vi "FPFA v4.vi"() -> ()   [LabVIEW 2015]
uses:
  <vilib>/Instr/_visa.llb/VISA Configure Serial Port (Instr).vi
  MFC1/inc/ThorZStepper.lvlib
panel:
  in  "Delay (s)":u32=1 min=1 step=1
  in  "# scan":u32=1 min=1 step=1
  in  "Autofocus":bool
  out "MFC1":bool
  out "Scan Enable":bool
  out "Current ZPos (mm)":dbl
  in  "Shutter":bool
  in  "MFC1 control":bool
  out "Scan finished":bool
  out "Elapsed Time (s)":dbl
  in  "# of measurment":i32=1
  out "Curr Well":cluster{"Row":u16, "Column":u16}={"Row"=1, "Column"=1} {"Column" items=["1", "2", "3", "4", "5", "6", "7", "8", "9", "10", "11", "12"]; "Row" items=["A", "B", "C", "D", "E", "F", "G", "H"]}
  in  "Set zero":bool
  in  "Abort":bool
  in  "Collection time":dbl=150.0 caption="s"
  in  "MoveWell":bool
  in  "Column":u16(ring)=1 items=["1", "2", "3", "4", "5", "6", "7", "8", "9", "10", "11", "12"]
  in  "Row":u16(ring)=1 items=["A", "B", "C", "D", "E", "F", "G", "H"]
  in  "Scan":bool
  in  "Move Abs":bool
  in  "YAbs":dbl caption="YAbs (micron)"
  in  "XAbs":dbl caption="XAbs (micron)"
  out "Response":string
  in  "Command":string
  out "error out":errorcluster
  in  "Send cmd":bool
  out "XPos":dbl
  out "YPos":dbl
  in  "Calibration":bool
  in  "stop":bool
  out "StageMoved":bool
  in  "Port":i32=5
  # "Move to Well"
  # "Stage Location"
  # "Move Absolute"
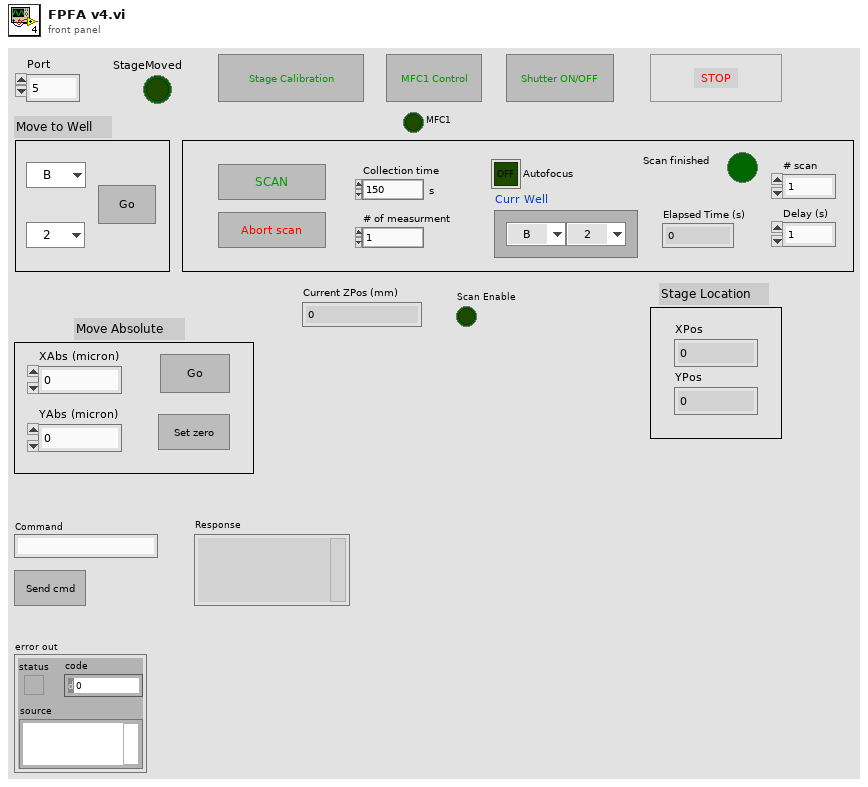
[diagram p1: front panel]
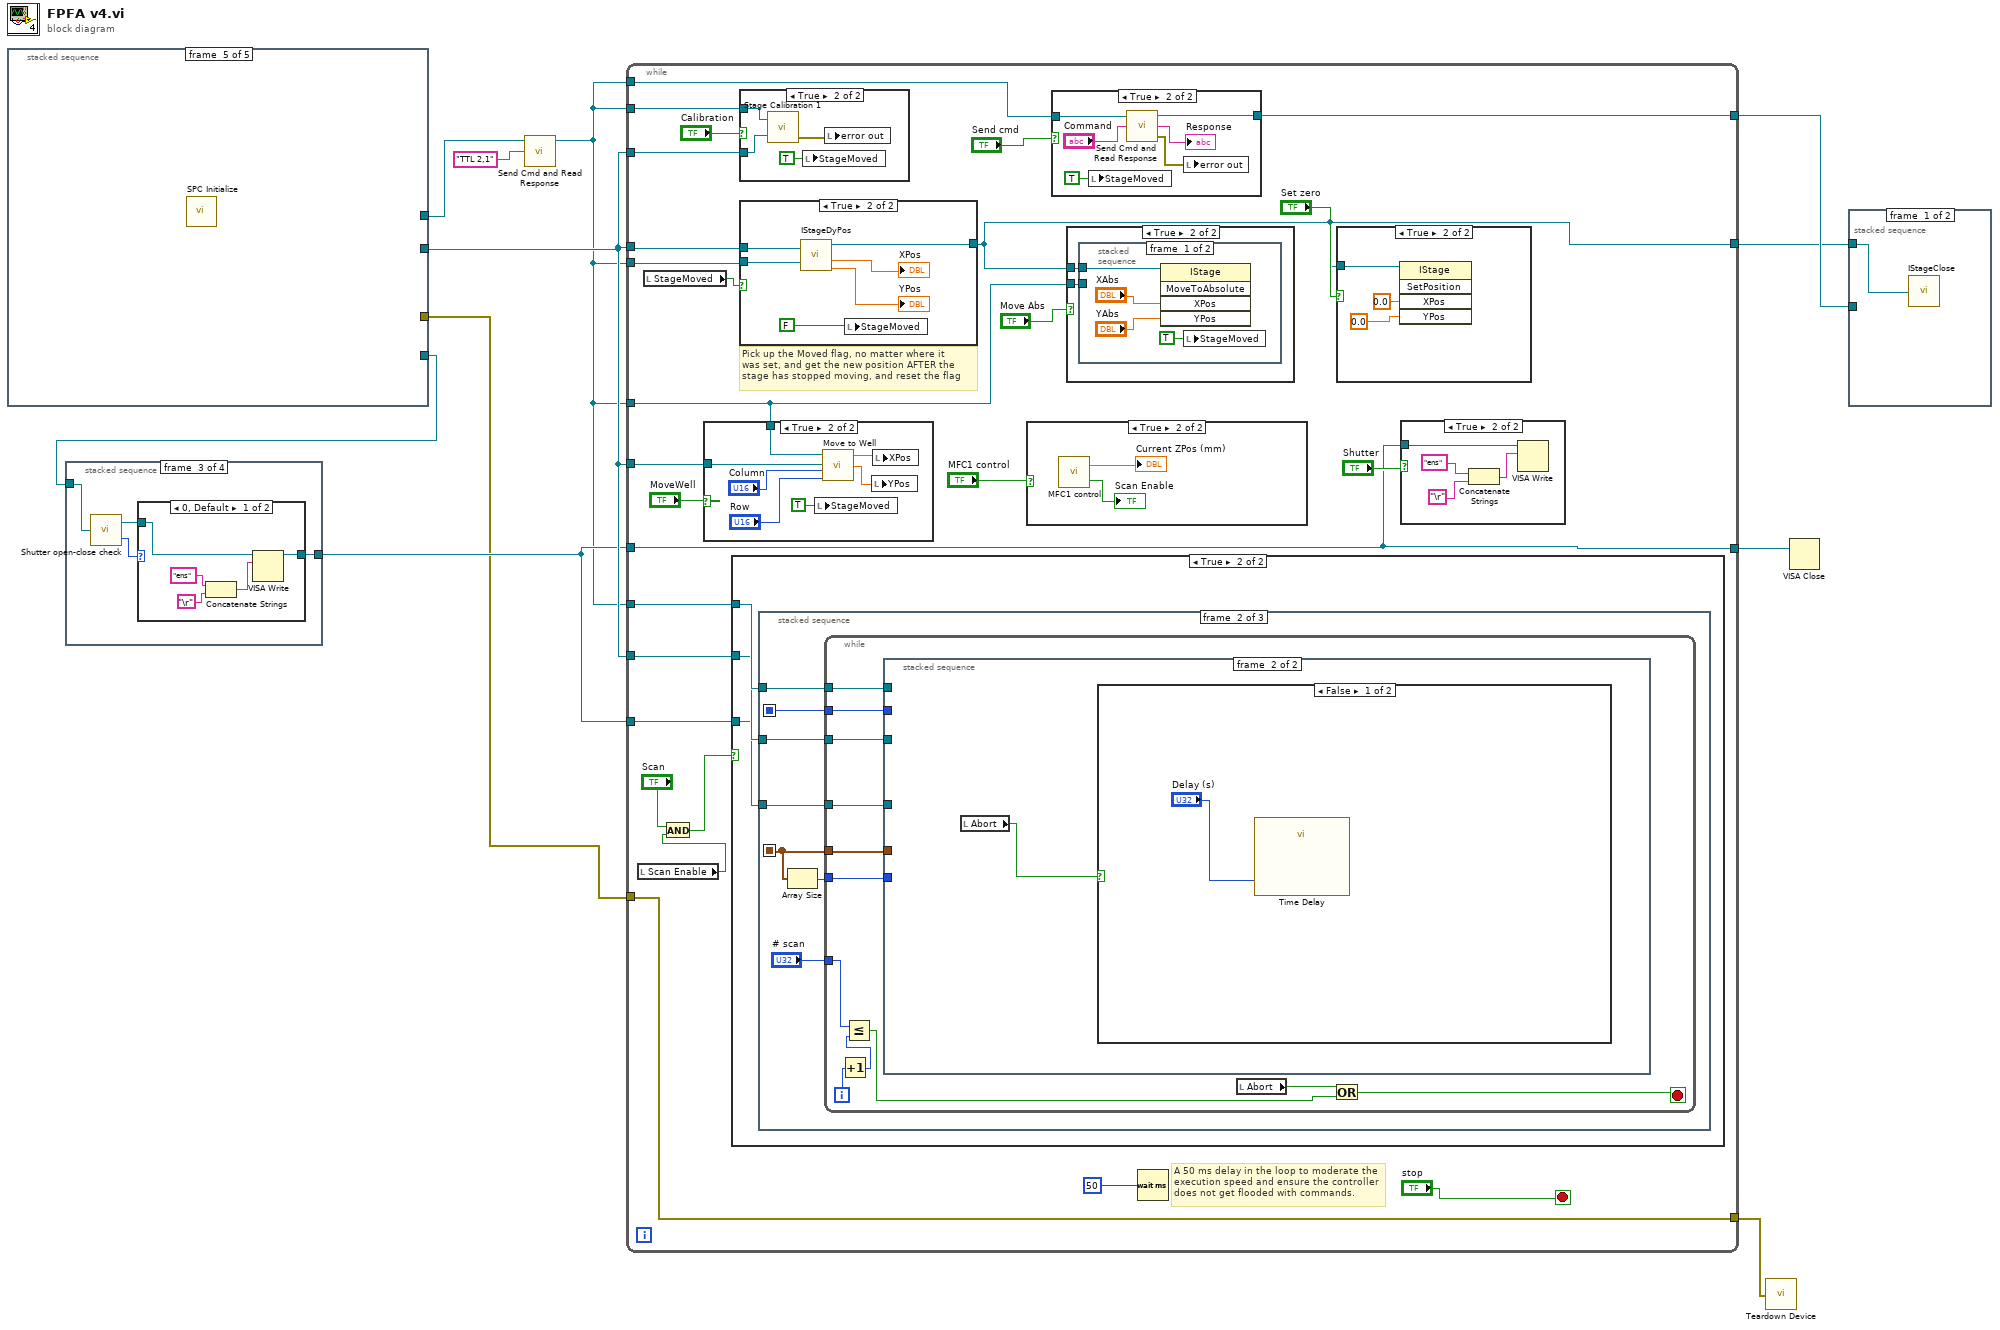
[diagram p0: block diagram]
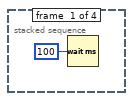
[diagram p2: hidden frame]
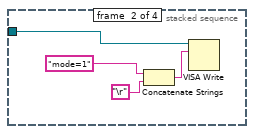
[diagram p3: hidden frame]
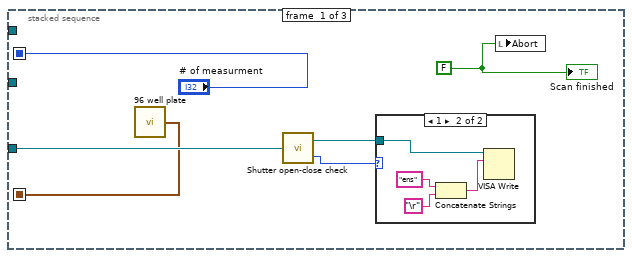
[diagram p10: hidden frame]
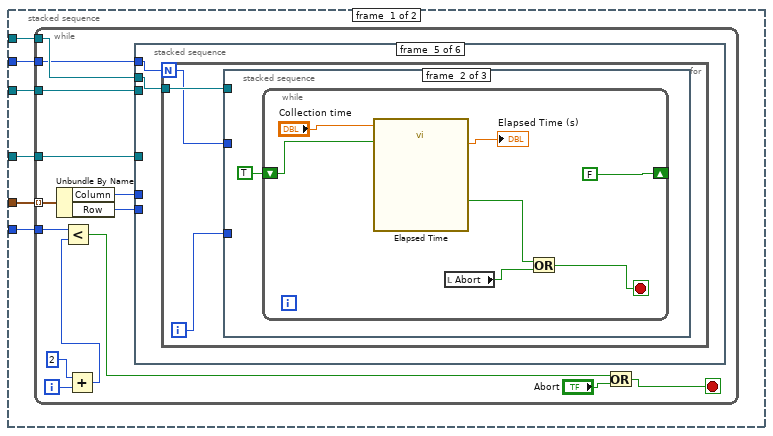
[diagram p12: hidden frame]
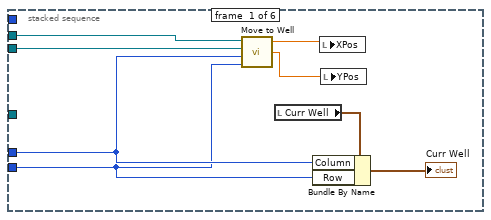
[diagram p13: hidden frame]
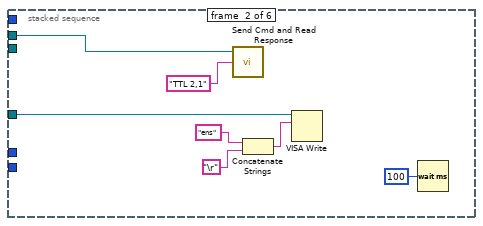
[diagram p14: hidden frame]
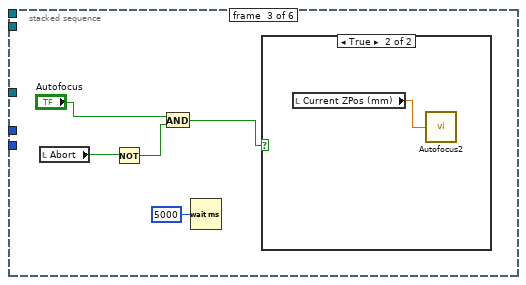
[diagram p15: hidden frame]
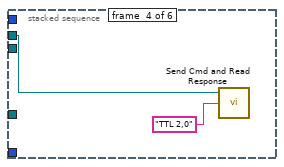
[diagram p17: hidden frame]
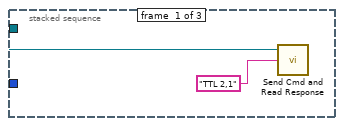
[diagram p18: hidden frame]
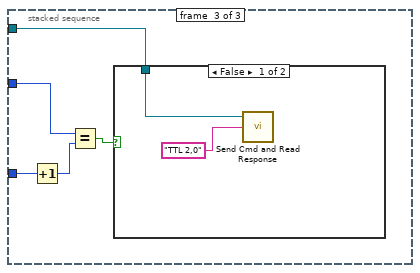
[diagram p19: hidden frame]
diagram:
  n1 = stacked-sequence {
    tunnel: [w13 _ _ _ _] -> w3
    tunnel: [_ w16 _ _ _] -> w9
    tunnel: [_ _ w17 _ _] -> w8
    tunnel: [_ _ _ w20 _] -> w1
    frame #0 {
      n2 = call "IScanOpen.vi"("Port"="Port") -> ("PRIORLib.IScanOut"=w13:refnum<k7>, "error out"=→"error out":errorcluster)  [unwired: 1 out]
      "StageMoved" <- TRUE
    }
    frame #1 {
      n3 = call "IStageOpen.vi"() -> ("PRIORLib.IStageOut"=w16:refnum<k7>)  [unwired: 1 in, 1 out]
    }
    frame #2 {
      n4 = call-poly "VISA Configure Serial Port"("VISA resource name"=refnum<visa-resource-name> "COM4", "Enable Termination\nChar (T)"=FALSE ("Enable Termination\nChar (T)")) -> ("VISA resource name out"=w17:refnum<visa-resource-name>)  [unwired: 12 in, 1 out]
    }
    frame #3 {
      n5 = call "Find Devices.vi"() -> ("function return"=w21:i32, "error out"=w22:errorcluster)  [unwired: 2 in, 1 out]
      n6 = case shown="1" w21 {
        tunnel: w22 -> [w23 w29]
        tunnel: [w23 w27] -> w20
        frame 0, Default {
        }
        frame 1 {
          n7 = call "Select Device.vi"("error in (no error)"=w29, "Device"=0) -> ("error out"=w27:errorcluster, "function return"=w25:i32)
          n8 = case shown="1" w25 {
            tunnel: [FALSE TRUE] -> w24
            frame 0, Default {
            }
            frame 1 {
              n9 = call "Move to new ZPos.vi"("New ZPos (mm)"=0.0) -> ("Current ZPos (mm)"=w31:dbl)  [unwired: 1 in, 1 out]
              n10 = local write "Current ZPos (mm)"(w31) -> ()
            }
          }
          "MFC1" <- w24
          n11 = call <vilib>:"Simple Error Handler.vi"("error in (no error)"=w27) -> ()  [unwired: 4 in, 5 out]
          n12 = local write "Scan Enable"(FALSE ("Autofocus Enable")) -> ()
        }
      }
    }
    frame #4 {
      n13 = call "SPC Initialize.vi"() -> ()  [unwired: 12 in]
    }
  }
  n14 = stacked-sequence {
    tunnel: w8 -> [_ w38 w42 _]
    tunnel: [_ _ w39 _] -> w7
    frame #0 {
      n15 = Wait (ms)(milliseconds to wait=u32 100) -> ()  [unwired: 1 out]
    }
    frame #1 {
      n16 = Concatenate Strings("mode=1", "\r") -> (w35:string)
      n17 = VISA Write(VISA resource name=w38, write buffer=w35) -> ()  [unwired: 1 in, 3 out]
    }
    frame #2 {
      n18 = call "Shutter open-close check.vi"("reference"=w42) -> ("VISA resource name out"=w40:refnum<visa-resource-name>, "number"=w41:i32)
      n19 = case shown="0, Default" w41 {
        tunnel: [w44 w48] -> w39
        tunnel: w40 -> [w43 w48]
        frame 0, Default {
          n20 = Concatenate Strings("ens", "\r") -> (w45:string)
          n21 = VISA Write(VISA resource name=w43, write buffer=w45) -> (VISA resource name out=w44:refnum<visa-resource-name>)  [unwired: 1 in, 2 out]
        }
        frame 1 {
        }
      }
    }
    frame #3 {
    }
  }
  n22 = call "Send Cmd and Read Response.vi"("cmd"="TTL 2,1", "PRIORLib.IScan"=w3) -> ("PRIORLib.IScanOut"=w2:refnum<k7>)  [unwired: 1 in, 2 out]
  n23 = while {
    tunnel: w2 -> [w74]
    tunnel: w9 -> [w69]
    tunnel: w2 -> [w70]
    tunnel: w2 -> [w67]
    tunnel: [w66] -> w11
    tunnel: [w57] -> w10
    tunnel: w9 -> [w65]
    tunnel: w2 -> [w61]
    tunnel: w9 -> [w63]
    tunnel: w9 -> [w60]
    tunnel: w2 -> [w59]
    tunnel: w7 -> [w56]
    tunnel: [w53] -> w6
    tunnel: w7 -> [w53]
    tunnel: [w55] -> w5
    tunnel: w1 -> [w55]
    stop <- "stop" stop-if-true
    # "Pick up the Moved flag, no matter where it\nwas set, and get the new position AFTER the\nstage has stopped moving, and reset the flag"
    # "A 50 ms delay in the loop to moderate the\nexecution speed and ensure the controller\ndoes not get flooded with commands."
    n24 = local read "Scan Enable"() -> (w52:bool)
    n25 = local read "StageMoved"() -> (w71:bool)
    n26 = And(x="Scan", y=w52) -> (x .and. y?=w50:bool)
    n27 = case shown="True" "MoveWell" {
      tunnel: w63 -> [_ w196]
      tunnel: w61 -> [_ w197]
      frame False {
      }
      frame True {
        n28 = local write "StageMoved"(TRUE ("StageMoved")) -> ()
        n29 = call "Move to Well.vi"("PRIORLib.IScan"=w197, "PRIORLib.IStage"=w196, "X"="Column", "Y"="Row") -> ("XPos"=w192:dbl, "YPos"=w191:dbl)  [unwired: 3 out]
        n30 = local write "YPos"(w191) -> ()
        n31 = local write "XPos"(w192) -> ()
      }
    }
    n32 = case shown="True" w50 {
      tunnel: w60 -> [_ w86]
      tunnel: w59 -> [_ w87]
      tunnel: w56 -> [_ w85]
      frame False {
      }
      frame True {
        n33 = stacked-sequence {
          seq-local: [w91 _ _] -> [_ w103 _]
          seq-local: ["# of measurment" _ _] -> [_ w99 _]
          tunnel: w87 -> [_ w102 _]
          tunnel: w86 -> [_ w101 _]
          tunnel: w85 -> [w92 w100 _]
          frame #0 {
            w88 = FALSE ("Abort")
            n34 = call "96 well plate.vi"() -> ("Selected wells"=w91:cluster{"Column":i32, "Row":i32}[])
            n35 = call "Shutter open-close check.vi"("reference"=w92) -> ("VISA resource name out"=w93:refnum<visa-resource-name>, "number"=w89:i32)
            n36 = case shown="1" w89 {
              tunnel: w93 -> [_ w94]
              frame 0, Default {
              }
              frame 1 {
                n37 = Concatenate Strings("ens", "\r") -> (w95:string)
                n38 = VISA Write(VISA resource name=w94, write buffer=w95) -> ()  [unwired: 1 in, 3 out]
              }
            }
            n39 = local write "Abort"(w88) -> ()
            "Scan finished" <- w88
          }
          frame #1 {
            n40 = Array Size(array=w103) -> (size(s)=w104:i32)
            n41 = while {
              tunnel: w104 -> [w116]
              tunnel: w103 -> [w115]
              tunnel: w102 -> [w114]
              tunnel: w101 -> [w113]
              tunnel: w100 -> [w112]
              tunnel: w99 -> [w111]
              tunnel: "# scan" -> [w110]
              i -> [w109]
              stop <- w105 stop-if-true
              n42 = Increment(x=w109) -> (x+1=w108:i32)
              n43 = Less Or Equal?(x=w110, y=w108) -> (x <= y?=w107:bool)
              n44 = stacked-sequence {
                tunnel: w116 -> [w122 _]
                tunnel: w115 -> [w121 _]
                tunnel: w114 -> [w120 _]
                tunnel: w113 -> [w119 _]
                tunnel: w112 -> [w118 _]
                tunnel: w111 -> [w117 _]
                frame #0 {
                  n45 = while {
                    tunnel: w122 -> [w134]
                    tunnel: w121 -> [w129] mode=indexing
                    tunnel: w120 -> [w128]
                    tunnel: w119 -> [w125]
                    tunnel: w118 -> [w124]
                    tunnel: w117 -> [w123]
                    i -> [w136]
                    stop <- w130 stop-if-true
                    n46 = Unbundle By Name(w129) -> ("Column"=w127:i32, "Row"=w126:i32)
                    n47 = Add(x=2, y=w136) -> (x+y=w133:i32)
                    n48 = Less?(x=w134, y=w133) -> (x < y?=w131:bool)
                    n49 = stacked-sequence {
                      tunnel: w128 -> [w144 w145 _ w158 w160 _]
                      tunnel: w127 -> [w138 _ _ _ _ _]
                      tunnel: w126 -> [w137 _ _ _ _ _]
                      tunnel: w125 -> [w143 _ _ _ _ _]
                      tunnel: w124 -> [_ w148 _ _ _ w183]
                      tunnel: w123 -> [_ _ _ _ w161 _]
                      frame #0 {
                        n50 = call "Move to Well.vi"("PRIORLib.IScan"=w144, "PRIORLib.IStage"=w143, "X"=w138, "Y"=w137) -> ("XPos"=w142:dbl, "YPos"=w141:dbl)  [unwired: 3 out]
                        n51 = local read "Curr Well"() -> (w140:cluster{"Row":u16, "Column":u16})
                        n52 = Bundle By Name(cluster=w140, "Column"=w138, "Row"=w137) -> (→"Curr Well":cluster{"Row":u16, "Column":u16})
                        n53 = local write "XPos"(w142) -> ()
                        n54 = local write "YPos"(w141) -> ()
                      }
                      frame #1 {
                        n55 = call "Send Cmd and Read Response.vi"("cmd"="TTL 2,1", "PRIORLib.IScan"=w145) -> ()  [unwired: 1 in, 3 out]
                        n56 = Concatenate Strings("ens", "\r") -> (w151:string)
                        n57 = VISA Write(VISA resource name=w148, write buffer=w151) -> ()  [unwired: 1 in, 3 out]
                        n58 = Wait (ms)(milliseconds to wait=u32 100) -> ()  [unwired: 1 out]
                      }
                      frame #2 {
                        n59 = local read "Abort"() -> (w156:bool)
                        n60 = Not(x=w156) -> (.not. x?=w154:bool)
                        n61 = And(x="Autofocus", y=w154) -> (x .and. y?=w153:bool)
                        n62 = Wait (ms)(milliseconds to wait=u32 5000) -> ()  [unwired: 1 out]
                        n63 = case shown="True" w153 {
                          frame False {
                          }
                          frame True {
                            n64 = local read "Current ZPos (mm)"() -> (w157:dbl)
                            n65 = call "Autofocus2.vi"("Set ZPos (mm)"=w157) -> ()  [unwired: 2 out]
                          }
                        }
                      }
                      frame #3 {
                        n66 = call "Send Cmd and Read Response.vi"("cmd"="TTL 2,0", "PRIORLib.IScan"=w158) -> ()  [unwired: 1 in, 3 out]
                      }
                      frame #4 {
                        n67 = for {
                          N: w161 -> [w163]
                          tunnel: w160 -> [w164]
                          i -> [w162]
                          n68 = stacked-sequence {
                            tunnel: w164 -> [w165 _ w177]
                            tunnel: w163 -> [_ _ w179]
                            tunnel: w162 -> [_ _ w176]
                            frame #0 {
                              n69 = call "Send Cmd and Read Response.vi"("cmd"="TTL 2,1", "PRIORLib.IScan"=w165) -> ()  [unwired: 1 in, 3 out]
                            }
                            frame #1 {
                              n70 = while {
                                shift-right: [FALSE] -> _
                                shift-left: TRUE -> [w170]
                                stop <- w172 stop-if-true
                                n71 = call "Elapsed Time"("Time Target (s)"="Collection time", "Reset"=w170) -> ("Elapsed Time (s)"=→"Elapsed Time (s)":dbl, "Time has Elapsed"=w171:bool)  [unwired: 10 in, 6 out]
                                n72 = local read "Abort"() -> (w173:bool)
                                n73 = Or(x=w171, y=w173) -> (x .or. y?=w172:bool)
                              }
                            }
                            frame #2 {
                              n74 = Increment(x=w176) -> (x+1=w175:i32)
                              n75 = Equal?(x=w179, y=w175) -> (x = y?=w178:bool)
                              n76 = case shown="False" w178 {
                                tunnel: w177 -> [w180 _]
                                frame False {
                                n77 = call "Send Cmd and Read Response.vi"("cmd"="TTL 2,0", "PRIORLib.IScan"=w180) -> ()  [unwired: 1 in, 3 out]
                                }
                                frame True {
                                }
                              }
                            }
                          }
                        }
                      }
                      frame #5 {
                        n78 = Concatenate Strings("ens", "\r") -> (w186:string)
                        n79 = VISA Write(VISA resource name=w183, write buffer=w186) -> ()  [unwired: 1 in, 3 out]
                        n80 = Wait (ms)(milliseconds to wait=u32 100) -> ()  [unwired: 1 out]
                      }
                    }
                    n81 = Or(x=w131, y="Abort") -> (x .or. y?=w130:bool)
                  }
                }
                frame #1 {
                  n82 = local read "Abort"() -> (w187:bool)
                  n83 = case shown="False" w187 {
                    frame False {
                      n84 = call "Time Delay"("Delay Time (s)"="Delay (s)") -> ()  [unwired: 10 in, 1 out]
                    }
                    frame True {
                    }
                  }
                }
              }
              n85 = local read "Abort"() -> (w106:bool)
              n86 = Or(x=w106, y=w107) -> (x .or. y?=w105:bool)
            }
          }
          frame #2 {
            n87 = local write "Scan finished"(TRUE) -> ()
            n88 = local write "Abort"(FALSE ("Abort")) -> ()
          }
        }
      }
    }
    n89 = case shown="True" "Calibration" {
      tunnel: w74 -> [_ w221]
      tunnel: w65 -> [_ w219]
      frame False {
      }
      frame True {
        n90 = call "Stage Calibration 1.vi"("PRIORLib.IScan"=w221, "PRIORLib.IStage"=w219) -> ("Error Out"=w222:errorcluster)  [unwired: 2 out]
        n91 = local write "StageMoved"(TRUE ("StageMoved")) -> ()
        n92 = local write "error out"(w222) -> ()
      }
    }
    n93 = case shown="True" w71 {
      tunnel: w69 -> [w212 w215]
      tunnel: w70 -> [_ w214]
      tunnel: [w212 w213] -> w57
      frame False {
      }
      frame True {
        n94 = call "IStageDyPos.vi"("PRIORLib.IStageIn"=w215, "PRIORLib.IScanIn"=w214) -> ("PRIORLib.IStageOut"=w213:refnum<k7>, "XPos"=→"XPos":dbl, "YPos"=→"YPos":dbl)  [unwired: 1 out]
        n95 = local write "StageMoved"(FALSE) -> ()
      }
    }
    n96 = case shown="True" "MFC1 control" {
      frame False {
      }
      frame True {
        n97 = call "MFC1 control.vi"() -> ("Autofocus Enable"=→"Scan Enable":bool, "Current ZPos (mm)"=→"Current ZPos (mm)":dbl)
      }
    }
    n98 = case shown="True" "Send cmd" {
      tunnel: w67 -> [w205 w211]
      tunnel: [w205 w210] -> w66
      frame False {
      }
      frame True {
        n99 = local write "StageMoved"(TRUE ("StageMoved")) -> ()
        n100 = call "Send Cmd and Read Response.vi"("cmd"="Command", "PRIORLib.IScan"=w211) -> ("error out"=w209:errorcluster, "String"=→"Response":string, "PRIORLib.IScanOut"=w210:refnum<k7>)  [unwired: 1 in]
        n101 = local write "error out"(w209) -> ()
      }
    }
    n102 = case shown="True" "Move Abs" {
      tunnel: w57 -> [_ w199]
      tunnel: w61 -> [_ w198]
      frame False {
      }
      frame True {
        n103 = stacked-sequence {
          tunnel: w199 -> [w203 _]
          tunnel: w198 -> [_ w204]
          frame #0 {
            n104 = invoke class="IStage" method="MoveToAbsolute"(reference=w203, "XPos"="XAbs", "YPos"="YAbs") -> ()  [unwired: 2 in, 5 out]
            n105 = local write "StageMoved"(TRUE ("StageMoved")) -> ()
          }
          frame #1 {
            n106 = call "Is Moving.vi"("PRIORLib.IScan"=w204) -> ()  [unwired: 1 in, 3 out]
          }
        }
      }
    }
    n107 = Wait (ms)(milliseconds to wait=u32 50) -> ()  [unwired: 1 out]
    n108 = case shown="True" "Set zero" {
      tunnel: w57 -> [_ w84]
      frame False {
      }
      frame True {
        n109 = invoke class="IStage" method="SetPosition"(reference=w84, "XPos"=0.0, "YPos"=0.0) -> ()  [unwired: 2 in, 5 out]
      }
    }
    n110 = case shown="True" "Shutter" {
      tunnel: w53 -> [_ w76]
      frame False {
      }
      frame True {
        n111 = Concatenate Strings("ens", "\r") -> (w77:string)
        n112 = VISA Write(VISA resource name=w76, write buffer=w77) -> ()  [unwired: 1 in, 3 out]
      }
    }
  }
  n113 = call "Teardown Device.vi"("error in (no error)"=w5) -> ()  [unwired: 2 out]
  n114 = VISA Close(VISA resource name=w6) -> ()  [unwired: 1 in, 1 out]
  n115 = stacked-sequence {
    tunnel: w11 -> [_ w224]
    tunnel: w10 -> [w223 _]
    frame #0 {
      n116 = call "IStageClose.vi"("PRIORLib.IStage"=w223) -> ()  [unwired: 1 out]
    }
    frame #1 {
      n117 = call "IScanClose.vi"("PRIORLib.IScan"=w224) -> ()  [unwired: 2 out]
    }
  }
